vi "Check FFMpeg.vi"(8 "error in (no error)":errorcluster, 11 "SB App in":refnum<class "SB App.lvclass">) -> (0 "error out":errorcluster, 3 "SB App out":refnum<class "SB App.lvclass">)   [LabVIEW 2020, in "SB App.lvlib" / "SB App.lvclass"]
uses:
  SB App.lvclass
  SB App.lvclass/SB App.ctl
  e423414c-d532-4016-b9a2-7a9e24746d79.vi
  6d728c5c-fc6a-4f37-8277-0cf76674c7fc.vi
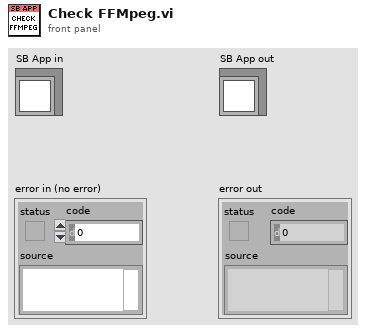
[diagram p1: front panel]
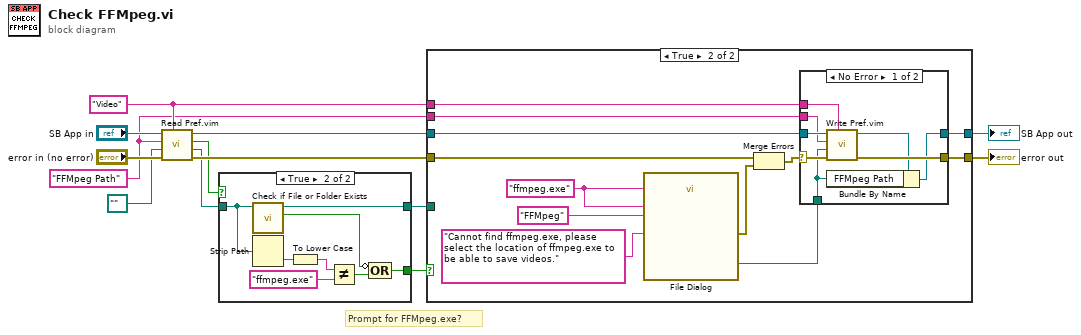
[diagram p0: block diagram]
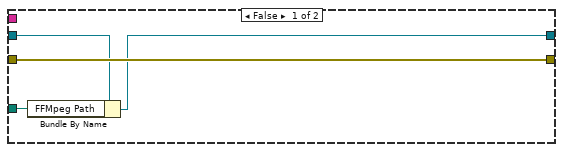
[diagram p2: hidden frame]
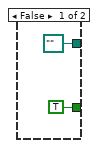
[diagram p4: hidden frame]
diagram:
  w1 = "FFMpeg Path" ("Key")
  w2 = "Video" ("Section")
  # "Prompt for FFMpeg.exe?"
  n1 = call "Read Pref.vim"("Section"=w2, "error in (no error)"="error in (no error)", "Type / Default (String)"=path "", "Key"=w1, "SB App in"="SB App in") -> ("error out"=w13:errorcluster, "value"=w8:path, "found?"=w9:bool, "SB App out"=w5:refnum<class "SB App.lvclass">)  [unwired: 3 in]
  n2 = case shown="True" w9 {
    tunnel: w8 -> [_ w20]
    tunnel: [path "" ("dup path") w17] -> w7
    tunnel: [TRUE w16] -> w6
    frame False {
    }
    frame True {
      n3 = call <vilib>:"Check if File or Folder Exists.vi"("path"=w20) -> ("file or folder exists?"=w19:bool, "dup path"=w17:path)  [unwired: 8 in, 1 out]
      n4 = Strip Path(path=w20) -> (name=w23:string)  [unwired: 1 out]
      n5 = To Lower Case(string=w23) -> (all lower case string=w22:string)
      n6 = Not Equal?(x=w22, y="ffmpeg.exe") -> (x != y?=w18:bool)
      n7 = Compound Arithmetic op=OR(invert w19, w18) -> (w16:bool)
    }
  }
  n8 = case shown="True" w6 {
    tunnel: w7 -> [w27 _]
    tunnel: w5 -> [w24 w32]
    tunnel: w13 -> [w26 w36]
    tunnel: [w26 w33] -> w4
    tunnel: [w25 w28] -> w3
    tunnel: w2 -> [_ w31]
    tunnel: w1 -> [_ w30]
    frame False {
      n9 = Bundle By Name(cluster=w24, "FFMpeg Path"=w27) -> (w25:refnum<class "SB App.lvclass">)
    }
    frame True {
      w39 = "ffmpeg.exe" ("default name")
      n10 = call "File Dialog"("prompt"="Cannot find ffmpeg.exe, please select the location of ffmpeg.exe to be able to save videos.", "default name"=w39, "pattern (all files)"=w39, "pattern label"="FFMpeg") -> ("selected path"=w29:path, "error out"=w35:errorcluster)  [unwired: 8 in, 2 out]
      n11 = Merge Errors(w36, w35) -> (w34:errorcluster)
      n12 = case shown="No Error" w34 {
        selector: w34 -> [w45 w49]
        tunnel: [w47 w49] -> w33
        tunnel: w32 -> [w46 w48]
        tunnel: w31 -> [w44 _]
        tunnel: w30 -> [w43 _]
        tunnel: w29 -> [w42 _]
        tunnel: [w40 w48] -> w28
        frame No Error {
          n13 = call "Write Pref.vim"("Section"=w44, "error in (no error)"=w45, "Value"=w42, "Key"=w43, "SB App in"=w46) -> ("error out"=w47:errorcluster, "SB App out"=w41:refnum<class "SB App.lvclass">)  [unwired: 5 in]
          n14 = Bundle By Name(cluster=w41, "FFMpeg Path"=w42) -> (w40:refnum<class "SB App.lvclass">)
        }
        frame Error {
        }
      }
    }
  }
  "error out" <- w4
  "SB App out" <- w3
